vi "update.type.request.vi"(8 "error in":errorcluster, 10 "Type":T1, 11 "event":refnum<class "event.lvclass">) -> (0 "error out":errorcluster, 3 "request":string)   [LabVIEW 2020, in "event.lvclass"]
uses:
  event.lvclass
  type.ctl
  event.lvclass/event.ctl
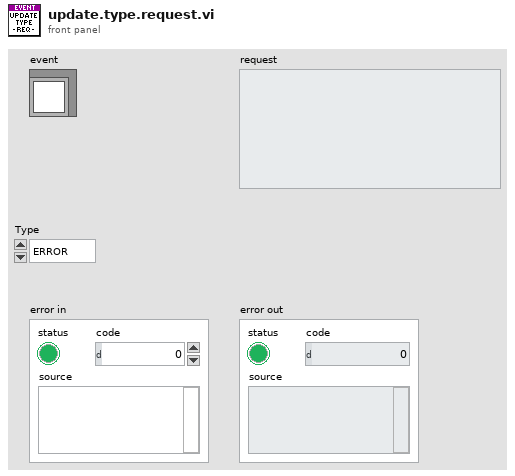
[diagram p1: front panel]
types:
  T1 = typedef "event.lvclass/type.ctl" = enum16{"ERROR", "FLAG", "INFO", "SUCCESS"}
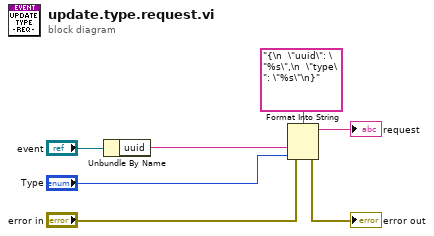
[diagram p0: block diagram]
diagram:
  n1 = Unbundle By Name("event") -> ("uuid"=w5:string)
  n2 = Format Into String(format string="{\n  \"uuid\": \"%s\",\n  \"type\": \"%s\"\n}", error in="error in", w5, "Type") -> (resulting string=→"request":string, error out=→"error out":errorcluster)  [unwired: 1 in]
